vi "Stop Target Actor.vi"(8 "error in":errorcluster, 11 "Study Actor in":refnum<class "Study Actor.lvclass">) -> (0 "error out":errorcluster, 3 "Study Actor out":refnum<class "Study Actor.lvclass">)   [LabVIEW 2023, in "Study Actor.lvlib" / "Study Actor.lvclass"]
uses:
  Study Actor.lvclass
  Study Actor.lvclass/Study Actor.ctl
  <vilib>/ActorFramework/Message Enqueuer/Message Enqueuer.lvclass/Message Enqueuer.ctl
  <vilib>/ActorFramework/Message Enqueuer/Enqueue.vi
  <vilib>/ActorFramework/Stop Msg/Stop Msg.lvclass
  C:/Program Files/National Instruments/LabVIEW 2023/vi.lib/ActorFramework/Message/Message.lvclass
  <vilib>/Utility/LVClass/Get LV Class Name.vi
  <resource>/AFDebug/Generate Trace for Message.vi
  <vilib>/ActorFramework/Message Priority Queue/Priority Enqueue.vi
  MSS Target/IMSS Target Actor Messages/Stop Target Actor Msg/Stop Target Actor Msg.lvclass
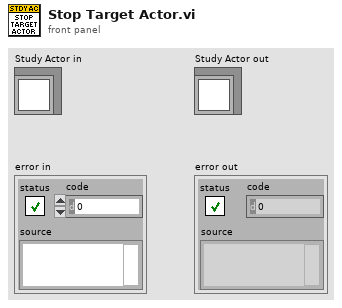
[diagram p1: front panel]
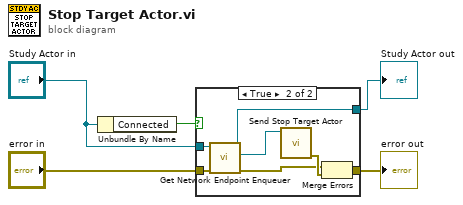
[diagram p0: block diagram]
diagram:
  n1 = Unbundle By Name("Study Actor in") -> ("Connected"=w2:bool)
  n2 = case shown="True" w2 {
    tunnel: "error in" -> [w7 w14]
    tunnel: "Study Actor in" -> [w6 w13]
    tunnel: [w6 w12] -> w4
    tunnel: [w7 w10] -> w3
    frame False {
    }
    frame True {
      n3 = call "Get Network Endpoint Enqueuer.vi"("error in"=w14, "Study Actor in"=w13) -> ("error out"=w8:errorcluster, "Network Endpoint Enqueuer"=w11:refnum<class "Message Enqueuer.lvclass">, "Study Actor out"=w12:refnum<class "Study Actor.lvclass">)  [unwired: 7 in]
      n4 = call "Send Stop Target Actor.vi"("Message Enqueuer"=w11) -> ("error out"=w9:errorcluster)  [unwired: 9 in, 1 out]
      n5 = Merge Errors(w8, w9) -> (w10:errorcluster)
    }
  }
  "error out" <- w3
  "Study Actor out" <- w4
